vi "ProcessingLoop.vi"(8 "error in (no error)":errorcluster, 11 "navX - Base in":refnum<class "navX - Interface.lvclass">) -> (0 "error out":errorcluster, 3 "navX - Base out":refnum<class "navX - Interface.lvclass">)   [LabVIEW 2015, in "navX Library v3.lvlib" / "navX - Interface.lvclass"]
uses:
  navX - Interface.lvclass
  navX Error Status/navX Error Status.lvclass
  navX - Interface.lvclass/navX - Interface.ctl
  <vilib>/Platform/TimedLoop/XDataNode/timing_clust.ctl
  <vilib>/Platform/TimedLoop/XDataNode/nitl_modes.ctl
  <vilib>/Platform/TimedLoop/XDataNode/wakeup.ctl
  <vilib>/platform/TimedLoop/XDataNode/XDataNode.xnode
  <vilib>/Platform/TimedLoop/XDataNode/XDNodeRunTimeDep.lvlib
panel:
  out "Iteration Duration":i64
  out "Finished Late? [i-1]":bool
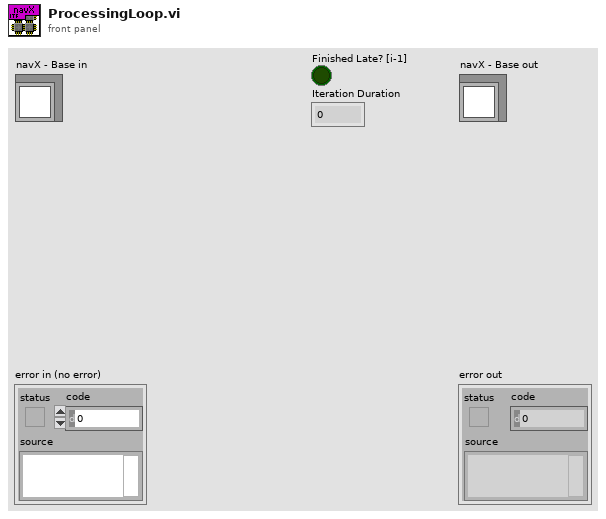
[diagram p1: front panel]
types:
  T1 = typedef "XDNodeRunTimeDep.lvlib/timing_clust.ctl" = cluster{"Expected End [f-1]":u64, "Actual End [f-1]":u64, "Finished Late? [f-1]":bool, "Expected End [i-1]":u64, "Actual End [i-1]":u64, "Finished Late? [i-1]":bool, "Expected Start [i]":u64, "Actual Start [i]":u64, "Expected Start [f]":u64, "Actual Start [f]":u64, "Source Name":string, "Structure Name":string, "Period":i64, "Deadline":i64, "Offset":i64, "Start":i64, "Priority":i32, "Timeout":i32, "Mode":T2, "Wakeup Reason":T3, "Error":errorcluster, "Source Type":string, "Secondary Source Type":string, "Global End Time":u64, "Global Start Time":u64, "Frame Duration":u64, "Iteration Duration":u64, "Assigned CPU":i32, "I/O Scan Engine Mode":u32}
  T2 = typedef "XDNodeRunTimeDep.lvlib/nitl_modes.ctl" = enum32{"No Change", "Process missed periods, maintain original phase", "Discard missed periods, maintain original phase", "Process missed periods, ignore original phase", "Discard missed periods, ignore original phase"}
  T3 = typedef "XDNodeRunTimeDep.lvlib/wakeup.ctl" = enum32{"Normal", "Aborted", "Asynchronous wakeup", "Timing source error", "Timed loop error", "Timeout"}
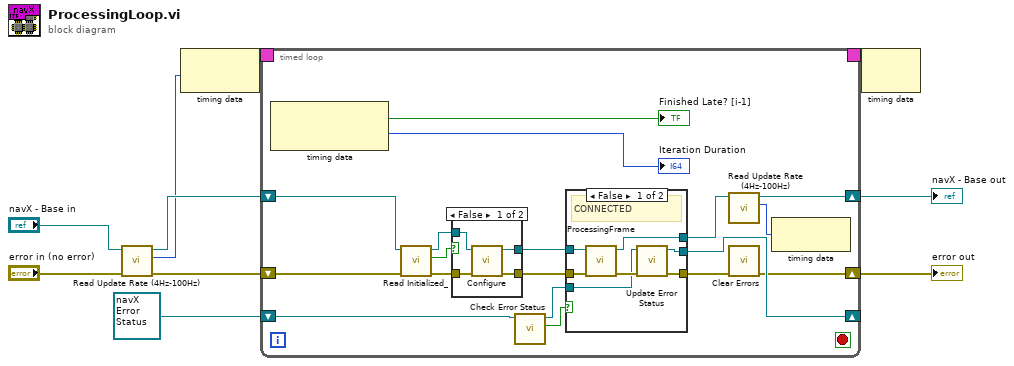
[diagram p0: block diagram]
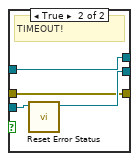
[diagram p3: hidden frame]
diagram:
  n1 = call "Read Update Rate (4Hz-100Hz).vi"("error in (no error)"="error in (no error)", "navX - Base in"="navX - Base in") -> ("error out"=w3:errorcluster, "Update Rate (4Hz-100Hz)"=w1:u8, "navX - Base out"=w4:refnum<class "navX - Interface.lvclass">)  [unwired: 7 in]
  n2 = node-c288(w1) -> (w6:T1)
  n3 = timed-loop {
    timing: w6 -> [_]
    timing-out: [_] -> w5
    shift-right: [w28] -> w7
    shift-left: w4 -> [w17]
    shift-right: [w20] -> w9
    shift-left: w3 -> [w16]
    shift-right: [w23] -> _
    shift-left: refnum<class "navX Error Status.lvclass"> refnum ("navX Library v3.lvlib:navX Error Status.lvclass") -> [w26]
    stop <- _ stop-if-true
    n4 = node-c288() -> (→"Finished Late? [i-1]":bool, →"Iteration Duration":i64)  [unwired: 1 in]
    n5 = call "Read Initialized_.vi"("error in (no error)"=w16, "navX - Base in"=w17) -> ("error out"=w13:errorcluster, "Initialized?"=w14:bool, "navX - Base out"=w15:refnum<class "navX - Interface.lvclass">)  [unwired: 7 in]
    n6 = case shown="False" w14 {
      tunnel: [w32 w33] -> w19
      tunnel: [w31 w34] -> w18
      tunnel: w15 -> [w30 w34]
      tunnel: w13 -> [w29 w33]
      frame False {
        n7 = call-dynamic "Configure.vi"("error in (no error)"=w29, "navX - Base in"=w30) -> ("error out"=w32:errorcluster, "navX - Base out"=w31:refnum<class "navX - Interface.lvclass">)  [unwired: 8 in]
      }
      frame True {
      }
    }
    n8 = call "Check Error Status.vi"("navX Error Status in"=w26) -> ("Timeout!"=w25:bool, "navX Error Status out"=w24:refnum<class "navX Error Status.lvclass">)  [unwired: 8 in, 1 out]
    n9 = case shown="False" w25 {
      tunnel: w24 -> [w38 w45]
      tunnel: w18 -> [w41 w43]
      tunnel: w19 -> [w40 w42]
      tunnel: [w37 w44] -> w23
      tunnel: [w36 w42] -> w21
      tunnel: [w35 w43] -> w22
      frame False {
        # "CONNECTED"
        n10 = call-dynamic "ProcessingFrame.vi"("error in (no error)"=w40, "navX - Base in"=w41) -> ("error out"=w39:errorcluster, "navX - Base out"=w35:refnum<class "navX - Interface.lvclass">)  [unwired: 8 in]
        n11 = call "Update Error Status.vi"("error in (no error)"=w39, "navX Status in"=w38) -> ("error out"=w36:errorcluster, "navX Status out"=w37:refnum<class "navX Error Status.lvclass">)  [unwired: 7 in, 1 out]
      }
      frame True {
        # "TIMEOUT!"
        n12 = call "Reset Error Status.vi"("navX Error Status in"=w45) -> ("navX Error Status out"=w44:refnum<class "navX Error Status.lvclass">)  [unwired: 9 in, 1 out]
      }
    }
    n13 = call "Read Update Rate (4Hz-100Hz).vi"("navX - Base in"=w22) -> ("Update Rate (4Hz-100Hz)"=w27:u8, "navX - Base out"=w28:refnum<class "navX - Interface.lvclass">)  [unwired: 8 in, 1 out]
    n14 = call <vilib>:"Clear Errors.vi"("error in (no error)"=w21) -> ("error out"=w20:errorcluster)  [unwired: 5 in, 1 out]
    n15 = node-c288(w27) -> ()  [unwired: 1 out]
  }
  "error out" <- w9
  "navX - Base out" <- w7
  n16 = node-c288(w5) -> ()  [unwired: 1 out]
